vi "Digital Clock.vi"() -> ()   [LabVIEW 2018]
panel:
  in  "1 unit = millisecond":u32
  out "Boolean 46":bool
  out "Boolean 45":bool
  out "Boolean 44":bool
  out "Boolean 43":bool
  out "Boolean 42":bool
  out "Boolean 41":bool
  out "Boolean 40":bool
  out "Boolean 39":bool
  out "Boolean 38":bool
  out "Boolean 37":bool
  out "Boolean 36":bool
  out "Boolean 35":bool
  out "Boolean 34":bool
  out "Boolean 33":bool
  out "Boolean 32":bool
  out "Boolean 31":bool
  out "Boolean 30":bool
  out "Boolean 29":bool
  out "Boolean 28":bool
  out "Boolean 27":bool
  out "Boolean 26":bool
  out "Boolean 25":bool
  out "Boolean 24":bool
  out "Boolean 23":bool
  out "Boolean 22":bool
  out "Boolean 21":bool
  out "Boolean 20":bool
  out "Boolean 19":bool
  out "Boolean 18":bool
  out "Boolean 17":bool
  out "Boolean 16":bool
  out "Boolean 15":bool
  out "Boolean 14":bool
  out "Boolean 13":bool
  out "Boolean 12":bool
  out "Boolean 11":bool
  out "Boolean 10":bool
  out "Boolean 9":bool
  out "Boolean 8":bool
  out "Boolean 7":bool
  out "Boolean 6":bool
  out "Boolean 5":bool
  out "Boolean 4":bool
  out "Boolean 3":bool
  out "Boolean 2":bool
  out "Boolean":bool
  # "HOURS"
  # "MINUTES"
  # "SECONDS"
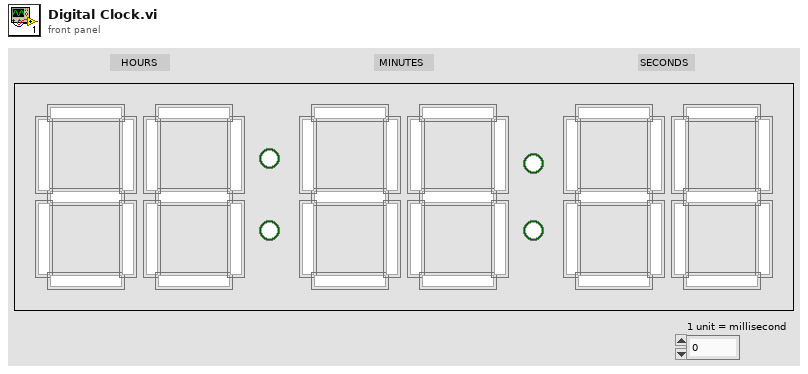
[diagram p1: front panel]
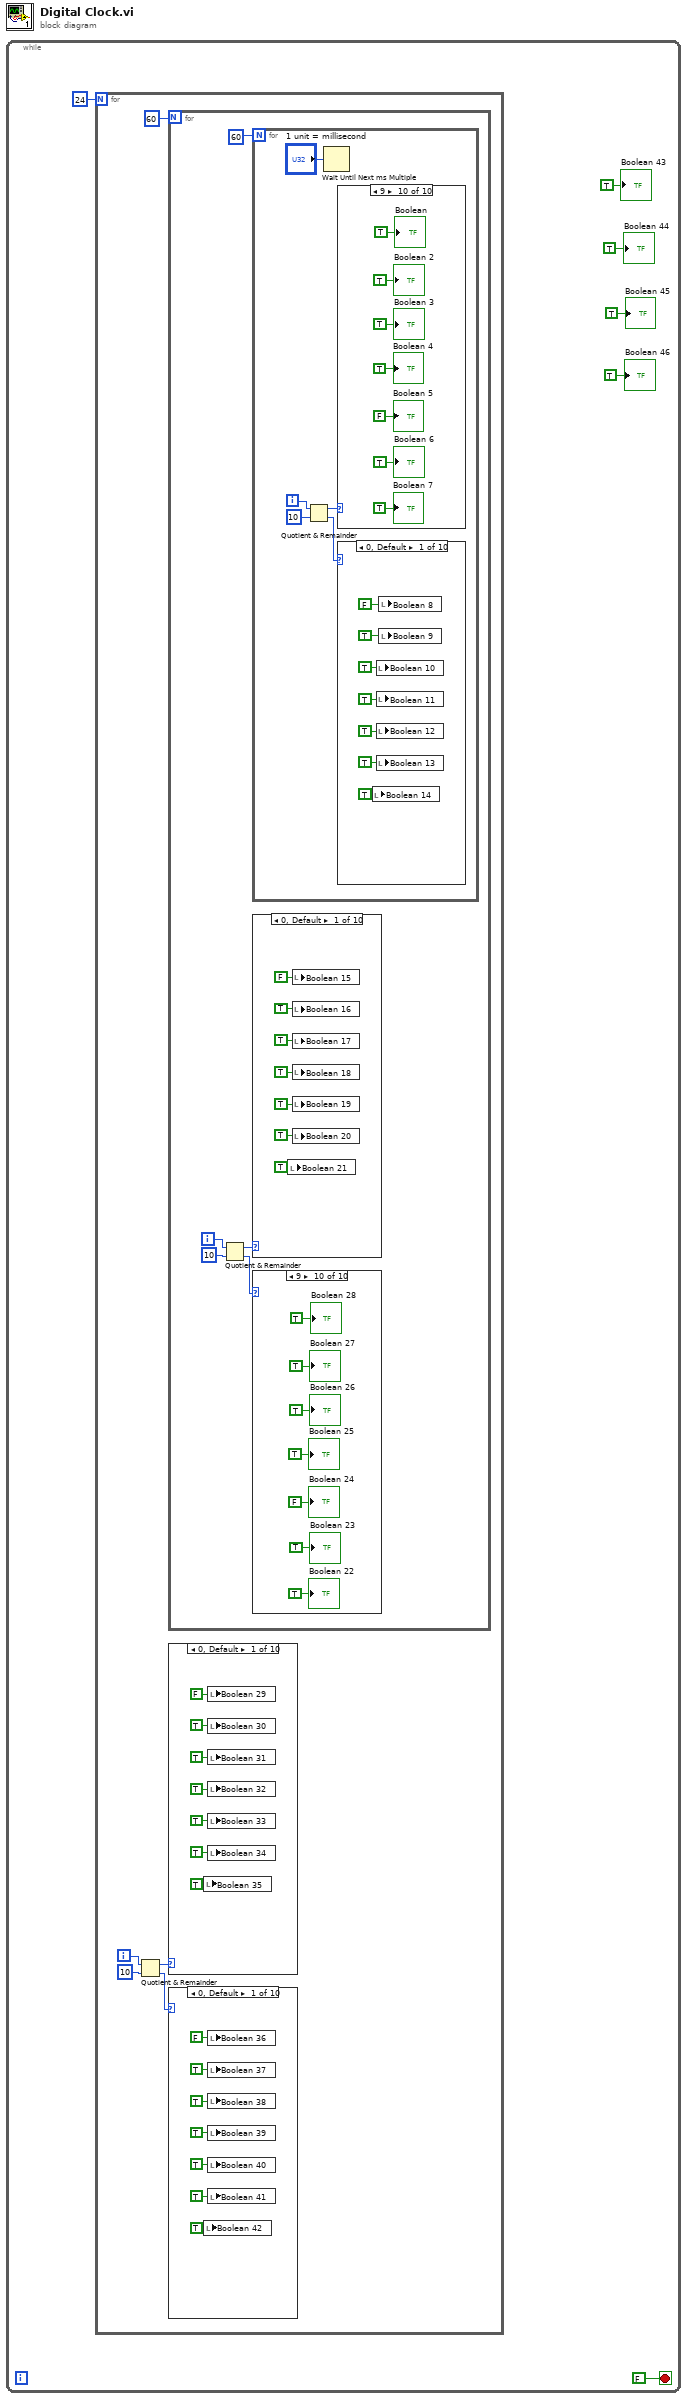
[diagram p0: block diagram]
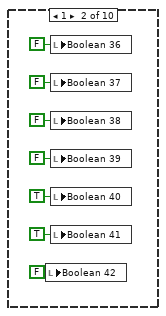
[diagram p2: hidden frame]
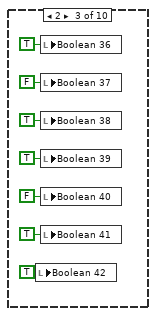
[diagram p3: hidden frame]
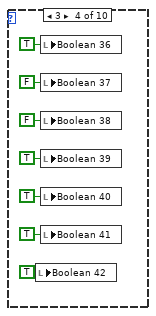
[diagram p4: hidden frame]
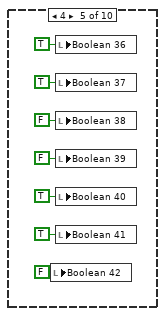
[diagram p5: hidden frame]
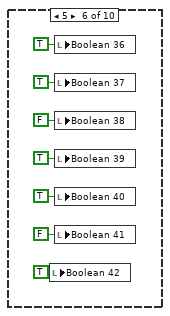
[diagram p6: hidden frame]
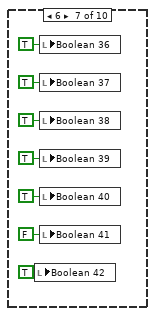
[diagram p7: hidden frame]
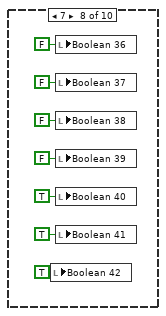
[diagram p8: hidden frame]
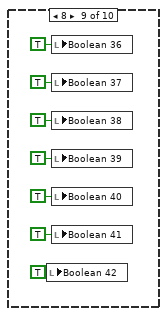
[diagram p9: hidden frame]
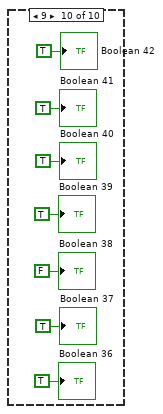
[diagram p10: hidden frame]
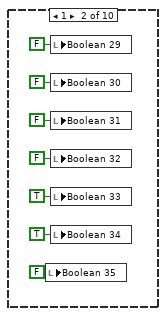
[diagram p11: hidden frame]
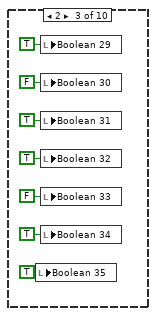
[diagram p12: hidden frame]
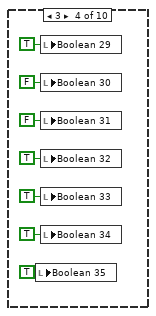
[diagram p13: hidden frame]
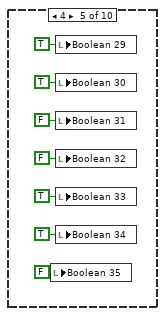
[diagram p14: hidden frame]
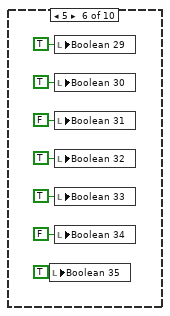
[diagram p15: hidden frame]
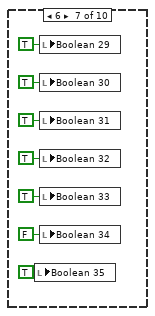
[diagram p16: hidden frame]
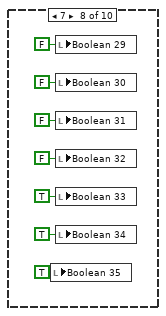
[diagram p17: hidden frame]
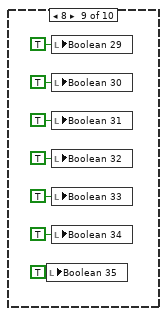
[diagram p18: hidden frame]
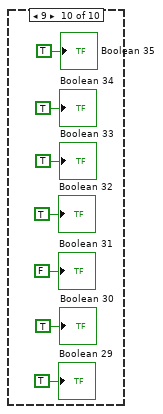
[diagram p19: hidden frame]
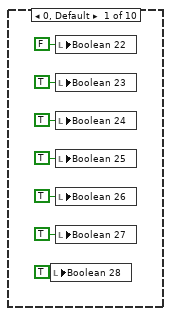
[diagram p20: hidden frame]
diagram:
  n1 = while {
    stop <- FALSE stop-if-true
    n2 = for {
      N: 24 -> [_]
      i -> [w10]
      n3 = Quotient & Remainder(x=w10, y=10) -> (x-y*floor(x/y)=w8:i32, floor(x/y)=w7:i32)
      n4 = for {
        N: 60 -> [_]
        i -> [w154]
        n5 = Quotient & Remainder(x=w154, y=10) -> (x-y*floor(x/y)=w155:i32, floor(x/y)=w152:i32)
        n6 = for {
          N: 60 -> [_]
          i -> [w301]
          n7 = Quotient & Remainder(x=w301, y=10) -> (x-y*floor(x/y)=w298:i32, floor(x/y)=w299:i32)
          n8 = Wait Until Next ms Multiple(millisecond multiple="1 unit = millisecond") -> ()  [unwired: 1 out]
          n9 = case shown="9" w298 {
            frame 0, Default {
              n10 = local write "Boolean 7"(FALSE ("Boolean 7")) -> ()
              n11 = local write "Boolean 6"(TRUE ("Boolean 6")) -> ()
              n12 = local write "Boolean 5"(TRUE ("Boolean 5")) -> ()
              n13 = local write "Boolean 4"(TRUE ("Boolean 4")) -> ()
              n14 = local write "Boolean 3"(TRUE ("Boolean 3")) -> ()
              n15 = local write "Boolean 2"(TRUE ("Boolean 2")) -> ()
              n16 = local write "Boolean"(TRUE ("Boolean")) -> ()
            }
            frame 1 {
              n17 = local write "Boolean 7"(FALSE ("Boolean 7")) -> ()
              n18 = local write "Boolean 6"(FALSE ("Boolean 6")) -> ()
              n19 = local write "Boolean 5"(FALSE ("Boolean 5")) -> ()
              n20 = local write "Boolean 4"(FALSE ("Boolean 4")) -> ()
              n21 = local write "Boolean 3"(TRUE ("Boolean 3")) -> ()
              n22 = local write "Boolean 2"(TRUE ("Boolean 2")) -> ()
              n23 = local write "Boolean"(FALSE ("Boolean")) -> ()
            }
            frame 2 {
              n24 = local write "Boolean 7"(TRUE ("Boolean 7")) -> ()
              n25 = local write "Boolean 6"(FALSE ("Boolean 6")) -> ()
              n26 = local write "Boolean 5"(TRUE ("Boolean 5")) -> ()
              n27 = local write "Boolean 4"(TRUE ("Boolean 4")) -> ()
              n28 = local write "Boolean 3"(FALSE ("Boolean 3")) -> ()
              n29 = local write "Boolean 2"(TRUE ("Boolean 2")) -> ()
              n30 = local write "Boolean"(TRUE ("Boolean")) -> ()
            }
            frame 3 {
              n31 = local write "Boolean 7"(TRUE ("Boolean 7")) -> ()
              n32 = local write "Boolean 6"(FALSE ("Boolean 6")) -> ()
              n33 = local write "Boolean 5"(FALSE ("Boolean 5")) -> ()
              n34 = local write "Boolean 4"(TRUE ("Boolean 4")) -> ()
              n35 = local write "Boolean 3"(TRUE ("Boolean 3")) -> ()
              n36 = local write "Boolean 2"(TRUE ("Boolean 2")) -> ()
              n37 = local write "Boolean"(TRUE ("Boolean")) -> ()
            }
            frame 4 {
              n38 = local write "Boolean 7"(TRUE ("Boolean 7")) -> ()
              n39 = local write "Boolean 6"(TRUE ("Boolean 6")) -> ()
              n40 = local write "Boolean 5"(FALSE ("Boolean 5")) -> ()
              n41 = local write "Boolean 4"(FALSE ("Boolean 4")) -> ()
              n42 = local write "Boolean 3"(TRUE ("Boolean 3")) -> ()
              n43 = local write "Boolean 2"(TRUE ("Boolean 2")) -> ()
              n44 = local write "Boolean"(FALSE ("Boolean")) -> ()
            }
            frame 5 {
              n45 = local write "Boolean 7"(TRUE ("Boolean 7")) -> ()
              n46 = local write "Boolean 6"(TRUE ("Boolean 6")) -> ()
              n47 = local write "Boolean 5"(FALSE ("Boolean 5")) -> ()
              n48 = local write "Boolean 4"(TRUE ("Boolean 4")) -> ()
              n49 = local write "Boolean 3"(TRUE ("Boolean 3")) -> ()
              n50 = local write "Boolean 2"(FALSE ("Boolean 2")) -> ()
              n51 = local write "Boolean"(TRUE ("Boolean")) -> ()
            }
            frame 6 {
              n52 = local write "Boolean 7"(TRUE ("Boolean 7")) -> ()
              n53 = local write "Boolean 6"(TRUE ("Boolean 6")) -> ()
              n54 = local write "Boolean 5"(TRUE ("Boolean 5")) -> ()
              n55 = local write "Boolean 4"(TRUE ("Boolean 4")) -> ()
              n56 = local write "Boolean 3"(TRUE ("Boolean 3")) -> ()
              n57 = local write "Boolean 2"(FALSE ("Boolean 2")) -> ()
              n58 = local write "Boolean"(TRUE ("Boolean")) -> ()
            }
            frame 7 {
              n59 = local write "Boolean 7"(FALSE ("Boolean 7")) -> ()
              n60 = local write "Boolean 6"(FALSE ("Boolean 6")) -> ()
              n61 = local write "Boolean 5"(FALSE ("Boolean 5")) -> ()
              n62 = local write "Boolean 4"(FALSE ("Boolean 4")) -> ()
              n63 = local write "Boolean 3"(TRUE ("Boolean 3")) -> ()
              n64 = local write "Boolean 2"(TRUE ("Boolean 2")) -> ()
              n65 = local write "Boolean"(TRUE ("Boolean")) -> ()
            }
            frame 8 {
              n66 = local write "Boolean 7"(TRUE ("Boolean 7")) -> ()
              n67 = local write "Boolean 6"(TRUE ("Boolean 6")) -> ()
              n68 = local write "Boolean 5"(TRUE ("Boolean 5")) -> ()
              n69 = local write "Boolean 4"(TRUE ("Boolean 4")) -> ()
              n70 = local write "Boolean 3"(TRUE ("Boolean 3")) -> ()
              n71 = local write "Boolean 2"(TRUE ("Boolean 2")) -> ()
              n72 = local write "Boolean"(TRUE ("Boolean")) -> ()
            }
            frame 9 {
              "Boolean" <- TRUE ("Boolean")
              "Boolean 2" <- TRUE ("Boolean 2")
              "Boolean 3" <- TRUE ("Boolean 3")
              "Boolean 4" <- TRUE ("Boolean 4")
              "Boolean 5" <- FALSE ("Boolean 5")
              "Boolean 6" <- TRUE ("Boolean 6")
              "Boolean 7" <- TRUE ("Boolean 7")
            }
          }
          n73 = case shown="0, Default" w299 {
            frame 0, Default {
              n74 = local write "Boolean 14"(TRUE ("Boolean")) -> ()
              n75 = local write "Boolean 10"(TRUE ("Boolean 5")) -> ()
              n76 = local write "Boolean 11"(TRUE ("Boolean 4")) -> ()
              n77 = local write "Boolean 12"(TRUE ("Boolean 3")) -> ()
              n78 = local write "Boolean 13"(TRUE ("Boolean 2")) -> ()
              n79 = local write "Boolean 8"(FALSE ("Boolean 7")) -> ()
              n80 = local write "Boolean 9"(TRUE ("Boolean 6")) -> ()
            }
            frame 1 {
              n81 = local write "Boolean 14"(FALSE ("Boolean")) -> ()
              n82 = local write "Boolean 10"(FALSE ("Boolean 5")) -> ()
              n83 = local write "Boolean 11"(FALSE ("Boolean 4")) -> ()
              n84 = local write "Boolean 12"(TRUE ("Boolean 3")) -> ()
              n85 = local write "Boolean 13"(TRUE ("Boolean 2")) -> ()
              n86 = local write "Boolean 8"(FALSE ("Boolean 7")) -> ()
              n87 = local write "Boolean 9"(FALSE ("Boolean 6")) -> ()
            }
            frame 2 {
              n88 = local write "Boolean 14"(TRUE ("Boolean")) -> ()
              n89 = local write "Boolean 10"(TRUE ("Boolean 5")) -> ()
              n90 = local write "Boolean 11"(TRUE ("Boolean 4")) -> ()
              n91 = local write "Boolean 12"(FALSE ("Boolean 3")) -> ()
              n92 = local write "Boolean 13"(TRUE ("Boolean 2")) -> ()
              n93 = local write "Boolean 8"(TRUE ("Boolean 7")) -> ()
              n94 = local write "Boolean 9"(FALSE ("Boolean 6")) -> ()
            }
            frame 3 {
              n95 = local write "Boolean 14"(TRUE ("Boolean")) -> ()
              n96 = local write "Boolean 10"(FALSE ("Boolean 5")) -> ()
              n97 = local write "Boolean 11"(TRUE ("Boolean 4")) -> ()
              n98 = local write "Boolean 12"(TRUE ("Boolean 3")) -> ()
              n99 = local write "Boolean 13"(TRUE ("Boolean 2")) -> ()
              n100 = local write "Boolean 8"(TRUE ("Boolean 7")) -> ()
              n101 = local write "Boolean 9"(FALSE ("Boolean 6")) -> ()
            }
            frame 4 {
              n102 = local write "Boolean 14"(FALSE ("Boolean")) -> ()
              n103 = local write "Boolean 10"(FALSE ("Boolean 5")) -> ()
              n104 = local write "Boolean 11"(FALSE ("Boolean 4")) -> ()
              n105 = local write "Boolean 12"(TRUE ("Boolean 3")) -> ()
              n106 = local write "Boolean 13"(TRUE ("Boolean 2")) -> ()
              n107 = local write "Boolean 8"(TRUE ("Boolean 7")) -> ()
              n108 = local write "Boolean 9"(TRUE ("Boolean 6")) -> ()
            }
            frame 5 {
              n109 = local write "Boolean 14"(TRUE ("Boolean")) -> ()
              n110 = local write "Boolean 10"(FALSE ("Boolean 5")) -> ()
              n111 = local write "Boolean 11"(TRUE ("Boolean 4")) -> ()
              n112 = local write "Boolean 12"(TRUE ("Boolean 3")) -> ()
              n113 = local write "Boolean 13"(FALSE ("Boolean 2")) -> ()
              n114 = local write "Boolean 8"(TRUE ("Boolean 7")) -> ()
              n115 = local write "Boolean 9"(TRUE ("Boolean 6")) -> ()
            }
            frame 6 {
              n116 = local write "Boolean 14"(TRUE ("Boolean")) -> ()
              n117 = local write "Boolean 10"(TRUE ("Boolean 5")) -> ()
              n118 = local write "Boolean 11"(TRUE ("Boolean 4")) -> ()
              n119 = local write "Boolean 12"(TRUE ("Boolean 3")) -> ()
              n120 = local write "Boolean 13"(FALSE ("Boolean 2")) -> ()
              n121 = local write "Boolean 8"(TRUE ("Boolean 7")) -> ()
              n122 = local write "Boolean 9"(TRUE ("Boolean 6")) -> ()
            }
            frame 7 {
              n123 = local write "Boolean 14"(TRUE ("Boolean")) -> ()
              n124 = local write "Boolean 10"(FALSE ("Boolean 5")) -> ()
              n125 = local write "Boolean 11"(FALSE ("Boolean 4")) -> ()
              n126 = local write "Boolean 12"(TRUE ("Boolean 3")) -> ()
              n127 = local write "Boolean 13"(TRUE ("Boolean 2")) -> ()
              n128 = local write "Boolean 8"(FALSE ("Boolean 7")) -> ()
              n129 = local write "Boolean 9"(FALSE ("Boolean 6")) -> ()
            }
            frame 8 {
              n130 = local write "Boolean 14"(TRUE ("Boolean")) -> ()
              n131 = local write "Boolean 10"(TRUE ("Boolean 5")) -> ()
              n132 = local write "Boolean 11"(TRUE ("Boolean 4")) -> ()
              n133 = local write "Boolean 12"(TRUE ("Boolean 3")) -> ()
              n134 = local write "Boolean 13"(TRUE ("Boolean 2")) -> ()
              n135 = local write "Boolean 8"(TRUE ("Boolean 7")) -> ()
              n136 = local write "Boolean 9"(TRUE ("Boolean 6")) -> ()
            }
            frame 9 {
              "Boolean 14" <- TRUE ("Boolean")
              "Boolean 13" <- TRUE ("Boolean 2")
              "Boolean 12" <- TRUE ("Boolean 3")
              "Boolean 11" <- TRUE ("Boolean 4")
              "Boolean 10" <- FALSE ("Boolean 5")
              "Boolean 9" <- TRUE ("Boolean 6")
              "Boolean 8" <- TRUE ("Boolean 7")
            }
          }
        }
        n137 = case shown="0, Default" w155 {
          frame 0, Default {
            n138 = local write "Boolean 21"(TRUE ("Boolean")) -> ()
            n139 = local write "Boolean 15"(FALSE ("Boolean 7")) -> ()
            n140 = local write "Boolean 16"(TRUE ("Boolean 6")) -> ()
            n141 = local write "Boolean 17"(TRUE ("Boolean 5")) -> ()
            n142 = local write "Boolean 18"(TRUE ("Boolean 4")) -> ()
            n143 = local write "Boolean 19"(TRUE ("Boolean 3")) -> ()
            n144 = local write "Boolean 20"(TRUE ("Boolean 2")) -> ()
          }
          frame 1 {
            n145 = local write "Boolean 21"(FALSE ("Boolean")) -> ()
            n146 = local write "Boolean 15"(FALSE ("Boolean 7")) -> ()
            n147 = local write "Boolean 16"(FALSE ("Boolean 6")) -> ()
            n148 = local write "Boolean 17"(FALSE ("Boolean 5")) -> ()
            n149 = local write "Boolean 18"(FALSE ("Boolean 4")) -> ()
            n150 = local write "Boolean 19"(TRUE ("Boolean 3")) -> ()
            n151 = local write "Boolean 20"(TRUE ("Boolean 2")) -> ()
          }
          frame 2 {
            n152 = local write "Boolean 21"(TRUE ("Boolean")) -> ()
            n153 = local write "Boolean 15"(TRUE ("Boolean 7")) -> ()
            n154 = local write "Boolean 16"(FALSE ("Boolean 6")) -> ()
            n155 = local write "Boolean 17"(TRUE ("Boolean 5")) -> ()
            n156 = local write "Boolean 18"(TRUE ("Boolean 4")) -> ()
            n157 = local write "Boolean 19"(FALSE ("Boolean 3")) -> ()
            n158 = local write "Boolean 20"(TRUE ("Boolean 2")) -> ()
          }
          frame 3 {
            n159 = local write "Boolean 21"(TRUE ("Boolean")) -> ()
            n160 = local write "Boolean 15"(TRUE ("Boolean 7")) -> ()
            n161 = local write "Boolean 16"(FALSE ("Boolean 6")) -> ()
            n162 = local write "Boolean 17"(FALSE ("Boolean 5")) -> ()
            n163 = local write "Boolean 18"(TRUE ("Boolean 4")) -> ()
            n164 = local write "Boolean 19"(TRUE ("Boolean 3")) -> ()
            n165 = local write "Boolean 20"(TRUE ("Boolean 2")) -> ()
          }
          frame 4 {
            n166 = local write "Boolean 21"(FALSE ("Boolean")) -> ()
            n167 = local write "Boolean 15"(TRUE ("Boolean 7")) -> ()
            n168 = local write "Boolean 16"(TRUE ("Boolean 6")) -> ()
            n169 = local write "Boolean 17"(FALSE ("Boolean 5")) -> ()
            n170 = local write "Boolean 18"(FALSE ("Boolean 4")) -> ()
            n171 = local write "Boolean 19"(TRUE ("Boolean 3")) -> ()
            n172 = local write "Boolean 20"(TRUE ("Boolean 2")) -> ()
          }
          frame 5 {
            n173 = local write "Boolean 21"(TRUE ("Boolean")) -> ()
            n174 = local write "Boolean 15"(TRUE ("Boolean 7")) -> ()
            n175 = local write "Boolean 16"(TRUE ("Boolean 6")) -> ()
            n176 = local write "Boolean 17"(FALSE ("Boolean 5")) -> ()
            n177 = local write "Boolean 18"(TRUE ("Boolean 4")) -> ()
            n178 = local write "Boolean 19"(TRUE ("Boolean 3")) -> ()
            n179 = local write "Boolean 20"(FALSE ("Boolean 2")) -> ()
          }
          frame 6 {
            n180 = local write "Boolean 21"(TRUE ("Boolean")) -> ()
            n181 = local write "Boolean 15"(TRUE ("Boolean 7")) -> ()
            n182 = local write "Boolean 16"(TRUE ("Boolean 6")) -> ()
            n183 = local write "Boolean 17"(TRUE ("Boolean 5")) -> ()
            n184 = local write "Boolean 18"(TRUE ("Boolean 4")) -> ()
            n185 = local write "Boolean 19"(TRUE ("Boolean 3")) -> ()
            n186 = local write "Boolean 20"(FALSE ("Boolean 2")) -> ()
          }
          frame 7 {
            n187 = local write "Boolean 21"(TRUE ("Boolean")) -> ()
            n188 = local write "Boolean 15"(FALSE ("Boolean 7")) -> ()
            n189 = local write "Boolean 16"(FALSE ("Boolean 6")) -> ()
            n190 = local write "Boolean 17"(FALSE ("Boolean 5")) -> ()
            n191 = local write "Boolean 18"(FALSE ("Boolean 4")) -> ()
            n192 = local write "Boolean 19"(TRUE ("Boolean 3")) -> ()
            n193 = local write "Boolean 20"(TRUE ("Boolean 2")) -> ()
          }
          frame 8 {
            n194 = local write "Boolean 21"(TRUE ("Boolean")) -> ()
            n195 = local write "Boolean 15"(TRUE ("Boolean 7")) -> ()
            n196 = local write "Boolean 16"(TRUE ("Boolean 6")) -> ()
            n197 = local write "Boolean 17"(TRUE ("Boolean 5")) -> ()
            n198 = local write "Boolean 18"(TRUE ("Boolean 4")) -> ()
            n199 = local write "Boolean 19"(TRUE ("Boolean 3")) -> ()
            n200 = local write "Boolean 20"(TRUE ("Boolean 2")) -> ()
          }
          frame 9 {
            "Boolean 21" <- TRUE ("Boolean")
            "Boolean 20" <- TRUE ("Boolean 2")
            "Boolean 19" <- TRUE ("Boolean 3")
            "Boolean 18" <- TRUE ("Boolean 4")
            "Boolean 17" <- FALSE ("Boolean 5")
            "Boolean 16" <- TRUE ("Boolean 6")
            "Boolean 15" <- TRUE ("Boolean 7")
          }
        }
        n201 = case shown="9" w152 {
          frame 0, Default {
            n202 = local write "Boolean 28"(TRUE ("Boolean")) -> ()
            n203 = local write "Boolean 22"(FALSE ("Boolean 7")) -> ()
            n204 = local write "Boolean 23"(TRUE ("Boolean 6")) -> ()
            n205 = local write "Boolean 24"(TRUE ("Boolean 5")) -> ()
            n206 = local write "Boolean 25"(TRUE ("Boolean 4")) -> ()
            n207 = local write "Boolean 26"(TRUE ("Boolean 3")) -> ()
            n208 = local write "Boolean 27"(TRUE ("Boolean 2")) -> ()
          }
          frame 1 {
            n209 = local write "Boolean 28"(FALSE ("Boolean")) -> ()
            n210 = local write "Boolean 22"(FALSE ("Boolean 7")) -> ()
            n211 = local write "Boolean 23"(FALSE ("Boolean 6")) -> ()
            n212 = local write "Boolean 24"(FALSE ("Boolean 5")) -> ()
            n213 = local write "Boolean 25"(FALSE ("Boolean 4")) -> ()
            n214 = local write "Boolean 26"(TRUE ("Boolean 3")) -> ()
            n215 = local write "Boolean 27"(TRUE ("Boolean 2")) -> ()
          }
          frame 2 {
            n216 = local write "Boolean 28"(TRUE ("Boolean")) -> ()
            n217 = local write "Boolean 22"(TRUE ("Boolean 7")) -> ()
            n218 = local write "Boolean 23"(FALSE ("Boolean 6")) -> ()
            n219 = local write "Boolean 24"(TRUE ("Boolean 5")) -> ()
            n220 = local write "Boolean 25"(TRUE ("Boolean 4")) -> ()
            n221 = local write "Boolean 26"(FALSE ("Boolean 3")) -> ()
            n222 = local write "Boolean 27"(TRUE ("Boolean 2")) -> ()
          }
          frame 3 {
            n223 = local write "Boolean 28"(TRUE ("Boolean")) -> ()
            n224 = local write "Boolean 22"(TRUE ("Boolean 7")) -> ()
            n225 = local write "Boolean 23"(FALSE ("Boolean 6")) -> ()
            n226 = local write "Boolean 24"(FALSE ("Boolean 5")) -> ()
            n227 = local write "Boolean 25"(TRUE ("Boolean 4")) -> ()
            n228 = local write "Boolean 26"(TRUE ("Boolean 3")) -> ()
            n229 = local write "Boolean 27"(TRUE ("Boolean 2")) -> ()
          }
          frame 4 {
            n230 = local write "Boolean 28"(FALSE ("Boolean")) -> ()
            n231 = local write "Boolean 22"(TRUE ("Boolean 7")) -> ()
            n232 = local write "Boolean 23"(TRUE ("Boolean 6")) -> ()
            n233 = local write "Boolean 24"(FALSE ("Boolean 5")) -> ()
            n234 = local write "Boolean 25"(FALSE ("Boolean 4")) -> ()
            n235 = local write "Boolean 26"(TRUE ("Boolean 3")) -> ()
            n236 = local write "Boolean 27"(TRUE ("Boolean 2")) -> ()
          }
          frame 5 {
            n237 = local write "Boolean 28"(TRUE ("Boolean")) -> ()
            n238 = local write "Boolean 22"(TRUE ("Boolean 7")) -> ()
            n239 = local write "Boolean 23"(TRUE ("Boolean 6")) -> ()
            n240 = local write "Boolean 24"(FALSE ("Boolean 5")) -> ()
            n241 = local write "Boolean 25"(TRUE ("Boolean 4")) -> ()
            n242 = local write "Boolean 26"(TRUE ("Boolean 3")) -> ()
            n243 = local write "Boolean 27"(FALSE ("Boolean 2")) -> ()
          }
          frame 6 {
            n244 = local write "Boolean 28"(TRUE ("Boolean")) -> ()
            n245 = local write "Boolean 22"(TRUE ("Boolean 7")) -> ()
            n246 = local write "Boolean 23"(TRUE ("Boolean 6")) -> ()
            n247 = local write "Boolean 24"(TRUE ("Boolean 5")) -> ()
            n248 = local write "Boolean 25"(TRUE ("Boolean 4")) -> ()
            n249 = local write "Boolean 26"(TRUE ("Boolean 3")) -> ()
            n250 = local write "Boolean 27"(FALSE ("Boolean 2")) -> ()
          }
          frame 7 {
            n251 = local write "Boolean 28"(TRUE ("Boolean")) -> ()
            n252 = local write "Boolean 22"(FALSE ("Boolean 7")) -> ()
            n253 = local write "Boolean 23"(FALSE ("Boolean 6")) -> ()
            n254 = local write "Boolean 24"(FALSE ("Boolean 5")) -> ()
            n255 = local write "Boolean 25"(FALSE ("Boolean 4")) -> ()
            n256 = local write "Boolean 26"(TRUE ("Boolean 3")) -> ()
            n257 = local write "Boolean 27"(TRUE ("Boolean 2")) -> ()
          }
          frame 8 {
            n258 = local write "Boolean 28"(TRUE ("Boolean")) -> ()
            n259 = local write "Boolean 22"(TRUE ("Boolean 7")) -> ()
            n260 = local write "Boolean 23"(TRUE ("Boolean 6")) -> ()
            n261 = local write "Boolean 24"(TRUE ("Boolean 5")) -> ()
            n262 = local write "Boolean 25"(TRUE ("Boolean 4")) -> ()
            n263 = local write "Boolean 26"(TRUE ("Boolean 3")) -> ()
            n264 = local write "Boolean 27"(TRUE ("Boolean 2")) -> ()
          }
          frame 9 {
            "Boolean 28" <- TRUE ("Boolean")
            "Boolean 27" <- TRUE ("Boolean 2")
            "Boolean 26" <- TRUE ("Boolean 3")
            "Boolean 25" <- TRUE ("Boolean 4")
            "Boolean 24" <- FALSE ("Boolean 5")
            "Boolean 23" <- TRUE ("Boolean 6")
            "Boolean 22" <- TRUE ("Boolean 7")
          }
        }
      }
      n265 = case shown="0, Default" w8 {
        frame 0, Default {
          n266 = local write "Boolean 35"(TRUE ("Boolean")) -> ()
          n267 = local write "Boolean 29"(FALSE ("Boolean 7")) -> ()
          n268 = local write "Boolean 30"(TRUE ("Boolean 6")) -> ()
          n269 = local write "Boolean 31"(TRUE ("Boolean 5")) -> ()
          n270 = local write "Boolean 32"(TRUE ("Boolean 4")) -> ()
          n271 = local write "Boolean 33"(TRUE ("Boolean 3")) -> ()
          n272 = local write "Boolean 34"(TRUE ("Boolean 2")) -> ()
        }
        frame 1 {
          n273 = local write "Boolean 35"(FALSE ("Boolean")) -> ()
          n274 = local write "Boolean 29"(FALSE ("Boolean 7")) -> ()
          n275 = local write "Boolean 30"(FALSE ("Boolean 6")) -> ()
          n276 = local write "Boolean 31"(FALSE ("Boolean 5")) -> ()
          n277 = local write "Boolean 32"(FALSE ("Boolean 4")) -> ()
          n278 = local write "Boolean 33"(TRUE ("Boolean 3")) -> ()
          n279 = local write "Boolean 34"(TRUE ("Boolean 2")) -> ()
        }
        frame 2 {
          n280 = local write "Boolean 35"(TRUE ("Boolean")) -> ()
          n281 = local write "Boolean 29"(TRUE ("Boolean 7")) -> ()
          n282 = local write "Boolean 30"(FALSE ("Boolean 6")) -> ()
          n283 = local write "Boolean 31"(TRUE ("Boolean 5")) -> ()
          n284 = local write "Boolean 32"(TRUE ("Boolean 4")) -> ()
          n285 = local write "Boolean 33"(FALSE ("Boolean 3")) -> ()
          n286 = local write "Boolean 34"(TRUE ("Boolean 2")) -> ()
        }
        frame 3 {
          n287 = local write "Boolean 35"(TRUE ("Boolean")) -> ()
          n288 = local write "Boolean 29"(TRUE ("Boolean 7")) -> ()
          n289 = local write "Boolean 30"(FALSE ("Boolean 6")) -> ()
          n290 = local write "Boolean 31"(FALSE ("Boolean 5")) -> ()
          n291 = local write "Boolean 32"(TRUE ("Boolean 4")) -> ()
          n292 = local write "Boolean 33"(TRUE ("Boolean 3")) -> ()
          n293 = local write "Boolean 34"(TRUE ("Boolean 2")) -> ()
        }
        frame 4 {
          n294 = local write "Boolean 35"(FALSE ("Boolean")) -> ()
          n295 = local write "Boolean 29"(TRUE ("Boolean 7")) -> ()
          n296 = local write "Boolean 30"(TRUE ("Boolean 6")) -> ()
          n297 = local write "Boolean 31"(FALSE ("Boolean 5")) -> ()
          n298 = local write "Boolean 32"(FALSE ("Boolean 4")) -> ()
          n299 = local write "Boolean 33"(TRUE ("Boolean 3")) -> ()
          n300 = local write "Boolean 34"(TRUE ("Boolean 2")) -> ()
        }
        frame 5 {
          n301 = local write "Boolean 35"(TRUE ("Boolean")) -> ()
          n302 = local write "Boolean 29"(TRUE ("Boolean 7")) -> ()
          n303 = local write "Boolean 30"(TRUE ("Boolean 6")) -> ()
          n304 = local write "Boolean 31"(FALSE ("Boolean 5")) -> ()
          n305 = local write "Boolean 32"(TRUE ("Boolean 4")) -> ()
          n306 = local write "Boolean 33"(TRUE ("Boolean 3")) -> ()
          n307 = local write "Boolean 34"(FALSE ("Boolean 2")) -> ()
        }
        frame 6 {
          n308 = local write "Boolean 35"(TRUE ("Boolean")) -> ()
          n309 = local write "Boolean 29"(TRUE ("Boolean 7")) -> ()
          n310 = local write "Boolean 30"(TRUE ("Boolean 6")) -> ()
          n311 = local write "Boolean 31"(TRUE ("Boolean 5")) -> ()
          n312 = local write "Boolean 32"(TRUE ("Boolean 4")) -> ()
          n313 = local write "Boolean 33"(TRUE ("Boolean 3")) -> ()
          n314 = local write "Boolean 34"(FALSE ("Boolean 2")) -> ()
        }
        frame 7 {
          n315 = local write "Boolean 35"(TRUE ("Boolean")) -> ()
          n316 = local write "Boolean 29"(FALSE ("Boolean 7")) -> ()
          n317 = local write "Boolean 30"(FALSE ("Boolean 6")) -> ()
          n318 = local write "Boolean 31"(FALSE ("Boolean 5")) -> ()
          n319 = local write "Boolean 32"(FALSE ("Boolean 4")) -> ()
          n320 = local write "Boolean 33"(TRUE ("Boolean 3")) -> ()
          n321 = local write "Boolean 34"(TRUE ("Boolean 2")) -> ()
        }
        frame 8 {
          n322 = local write "Boolean 35"(TRUE ("Boolean")) -> ()
          n323 = local write "Boolean 29"(TRUE ("Boolean 7")) -> ()
          n324 = local write "Boolean 30"(TRUE ("Boolean 6")) -> ()
          n325 = local write "Boolean 31"(TRUE ("Boolean 5")) -> ()
          n326 = local write "Boolean 32"(TRUE ("Boolean 4")) -> ()
          n327 = local write "Boolean 33"(TRUE ("Boolean 3")) -> ()
          n328 = local write "Boolean 34"(TRUE ("Boolean 2")) -> ()
        }
        frame 9 {
          "Boolean 35" <- TRUE ("Boolean")
          "Boolean 34" <- TRUE ("Boolean 2")
          "Boolean 33" <- TRUE ("Boolean 3")
          "Boolean 32" <- TRUE ("Boolean 4")
          "Boolean 31" <- FALSE ("Boolean 5")
          "Boolean 30" <- TRUE ("Boolean 6")
          "Boolean 29" <- TRUE ("Boolean 7")
        }
      }
      n329 = case shown="0, Default" w7 {
        frame 0, Default {
          n330 = local write "Boolean 42"(TRUE ("Boolean")) -> ()
          n331 = local write "Boolean 36"(FALSE ("Boolean 7")) -> ()
          n332 = local write "Boolean 37"(TRUE ("Boolean 6")) -> ()
          n333 = local write "Boolean 38"(TRUE ("Boolean 5")) -> ()
          n334 = local write "Boolean 39"(TRUE ("Boolean 4")) -> ()
          n335 = local write "Boolean 40"(TRUE ("Boolean 3")) -> ()
          n336 = local write "Boolean 41"(TRUE ("Boolean 2")) -> ()
        }
        frame 1 {
          n337 = local write "Boolean 42"(FALSE ("Boolean")) -> ()
          n338 = local write "Boolean 36"(FALSE ("Boolean 7")) -> ()
          n339 = local write "Boolean 37"(FALSE ("Boolean 6")) -> ()
          n340 = local write "Boolean 38"(FALSE ("Boolean 5")) -> ()
          n341 = local write "Boolean 39"(FALSE ("Boolean 4")) -> ()
          n342 = local write "Boolean 40"(TRUE ("Boolean 3")) -> ()
          n343 = local write "Boolean 41"(TRUE ("Boolean 2")) -> ()
        }
        frame 2 {
          n344 = local write "Boolean 42"(TRUE ("Boolean")) -> ()
          n345 = local write "Boolean 36"(TRUE ("Boolean 7")) -> ()
          n346 = local write "Boolean 37"(FALSE ("Boolean 6")) -> ()
          n347 = local write "Boolean 38"(TRUE ("Boolean 5")) -> ()
          n348 = local write "Boolean 39"(TRUE ("Boolean 4")) -> ()
          n349 = local write "Boolean 40"(FALSE ("Boolean 3")) -> ()
          n350 = local write "Boolean 41"(TRUE ("Boolean 2")) -> ()
        }
        frame 3 {
          n351 = local write "Boolean 42"(TRUE ("Boolean")) -> ()
          n352 = local write "Boolean 36"(TRUE ("Boolean 7")) -> ()
          n353 = local write "Boolean 37"(FALSE ("Boolean 6")) -> ()
          n354 = local write "Boolean 38"(FALSE ("Boolean 5")) -> ()
          n355 = local write "Boolean 39"(TRUE ("Boolean 4")) -> ()
          n356 = local write "Boolean 40"(TRUE ("Boolean 3")) -> ()
          n357 = local write "Boolean 41"(TRUE ("Boolean 2")) -> ()
        }
        frame 4 {
          n358 = local write "Boolean 42"(FALSE ("Boolean")) -> ()
          n359 = local write "Boolean 36"(TRUE ("Boolean 7")) -> ()
          n360 = local write "Boolean 37"(TRUE ("Boolean 6")) -> ()
          n361 = local write "Boolean 38"(FALSE ("Boolean 5")) -> ()
          n362 = local write "Boolean 39"(FALSE ("Boolean 4")) -> ()
          n363 = local write "Boolean 40"(TRUE ("Boolean 3")) -> ()
          n364 = local write "Boolean 41"(TRUE ("Boolean 2")) -> ()
        }
        frame 5 {
          n365 = local write "Boolean 42"(TRUE ("Boolean")) -> ()
          n366 = local write "Boolean 36"(TRUE ("Boolean 7")) -> ()
          n367 = local write "Boolean 37"(TRUE ("Boolean 6")) -> ()
          n368 = local write "Boolean 38"(FALSE ("Boolean 5")) -> ()
          n369 = local write "Boolean 39"(TRUE ("Boolean 4")) -> ()
          n370 = local write "Boolean 40"(TRUE ("Boolean 3")) -> ()
          n371 = local write "Boolean 41"(FALSE ("Boolean 2")) -> ()
        }
        frame 6 {
          n372 = local write "Boolean 42"(TRUE ("Boolean")) -> ()
          n373 = local write "Boolean 36"(TRUE ("Boolean 7")) -> ()
          n374 = local write "Boolean 37"(TRUE ("Boolean 6")) -> ()
          n375 = local write "Boolean 38"(TRUE ("Boolean 5")) -> ()
          n376 = local write "Boolean 39"(TRUE ("Boolean 4")) -> ()
          n377 = local write "Boolean 40"(TRUE ("Boolean 3")) -> ()
          n378 = local write "Boolean 41"(FALSE ("Boolean 2")) -> ()
        }
        frame 7 {
          n379 = local write "Boolean 42"(TRUE ("Boolean")) -> ()
          n380 = local write "Boolean 36"(FALSE ("Boolean 7")) -> ()
          n381 = local write "Boolean 37"(FALSE ("Boolean 6")) -> ()
          n382 = local write "Boolean 38"(FALSE ("Boolean 5")) -> ()
          n383 = local write "Boolean 39"(FALSE ("Boolean 4")) -> ()
          n384 = local write "Boolean 40"(TRUE ("Boolean 3")) -> ()
          n385 = local write "Boolean 41"(TRUE ("Boolean 2")) -> ()
        }
        frame 8 {
          n386 = local write "Boolean 42"(TRUE ("Boolean")) -> ()
          n387 = local write "Boolean 36"(TRUE ("Boolean 7")) -> ()
          n388 = local write "Boolean 37"(TRUE ("Boolean 6")) -> ()
          n389 = local write "Boolean 38"(TRUE ("Boolean 5")) -> ()
          n390 = local write "Boolean 39"(TRUE ("Boolean 4")) -> ()
          n391 = local write "Boolean 40"(TRUE ("Boolean 3")) -> ()
          n392 = local write "Boolean 41"(TRUE ("Boolean 2")) -> ()
        }
        frame 9 {
          "Boolean 42" <- TRUE ("Boolean")
          "Boolean 41" <- TRUE ("Boolean 2")
          "Boolean 40" <- TRUE ("Boolean 3")
          "Boolean 39" <- TRUE ("Boolean 4")
          "Boolean 38" <- FALSE ("Boolean 5")
          "Boolean 37" <- TRUE ("Boolean 6")
          "Boolean 36" <- TRUE ("Boolean 7")
        }
      }
    }
    "Boolean 43" <- TRUE ("Boolean 43")
    "Boolean 44" <- TRUE ("Boolean 44")
    "Boolean 45" <- TRUE ("Boolean 45")
    "Boolean 46" <- TRUE ("Boolean 46")
  }
